vi "GUI Main Window.vi"() -> ()   [LabVIEW 2011]
doc: "Fast Orbit Feedback (FOFB) graphical user interface."
uses:
  Types Definitions/Type Configuration Loop Mode.ctl
  <vilib>/Platform/TimedLoop/XDataNode/timing_clust.ctl
  <vilib>/Platform/TimedLoop/XDataNode/nitl_modes.ctl
  <vilib>/Platform/TimedLoop/XDataNode/wakeup.ctl
  Types Definitions/Type Diagnostics Sample.ctl
  Types Definitions/Type Diagnostics Data.ctl
  Types Definitions/Type CPU Loads Array.ctl
  Types Definitions/Type CPU Loads.ctl
  Types Definitions/Type Monitoring Sample.ctl
  Types Definitions/Type FOFB Parameters.ctl
  Types Definitions/Type Network Configuration.ctl
  Types Definitions/Type FA Configuration.ctl
  Types Definitions/Type Response Matrix Measurement Configuration.ctl
  Types Definitions/Type Correction Algorithm Configuration.ctl
  Types Definitions/Type Acquisition Network Configuration.ctl
  Types Definitions/Type Actuation Network Configuration.ctl
  Types Definitions/Type BPM or PS Selector.ctl
  <vilib>/Analysis/5stat.llb/RMS (DBL).vi
  GUI Monitoring Graph Selection Window.vi
  <vilib>/Platform/TimedLoop/XDataNode/XDataNode.xnode
  <vilib>/Platform/TimedLoop/XDataNode/XDNodeRunTimeDep.lvlib
  File VIs.lvlib
  Type Definitions.lvlib
  Third Party/bean/bean.lvlib
  User Interface Window VIs.lvlib
  User Interface VIs.lvlib
  XML VIs.lvlib
  Filter VIs.lvlib
  <vilib>/Analysis/NI_AALPro.lvlib
panel:
  out "error out":errorcluster
  out "Connected":bool
  in  "Open Computer Performance":bool
  in  "Open BPM RMS/Min/Max Monitoring Graph":bool
  out "Orbit Path":path caption="Endereço da Órbita de Referência"
  in  "Open Configuration GUI":bool
  in  "Max Scale Y":dbl=1.0 min=0.001 max=20.0 format="%6.3g"
  in  "Max Scale X":dbl=1.0 min=0.001 max=20.0 format="%6.3g"
  in  "Auto-Scale":bool
  in  "Open BPM-PS Monitoring Graph":bool
  out "Reference Orbit":dbl[](array[numeric])
  in  "Orbit Source":enum32{"Zero", "From File", "Current Orbit"}(radio)
  out "Current Orbit":dbl[](array[numeric])
  out "Operation Mode (Controller to GUI)":T1(ring) caption="Modo de Operação"
  in  "Send Orbit":bool
  out "Min Y @":string="AMP05A" caption="@"
  out "MaxY @":string="AMP05A" caption="@"
  out "RMS Y":dbl=-1.1111 caption="RMS =" format="%#.4g"
  out "Min Y":dbl=-1.2564 caption="Min =" format="%#.4g"
  out "Max. Y":dbl=1.1111 caption="Max =" format="%#.4g"
  out "Min X @":string="AMP01A" caption="@"
  out "Max X @":string="AMP01A" caption="@"
  out "RMS X":dbl=21.1111 caption="RMS =" format="%#.4g"
  out "Min X":dbl=1.1111 caption="Min =" format="%#.4g"
  out "Max. X":dbl=1.1111 caption="Max =" format="%#.4g"
  out "Horizontal":cluster{i32, dbl}[](graph)
  out "Vertical":cluster{i32, dbl}[](graph)
  in  "Save Orbit":bool
  # "Órbita de Referência Local"
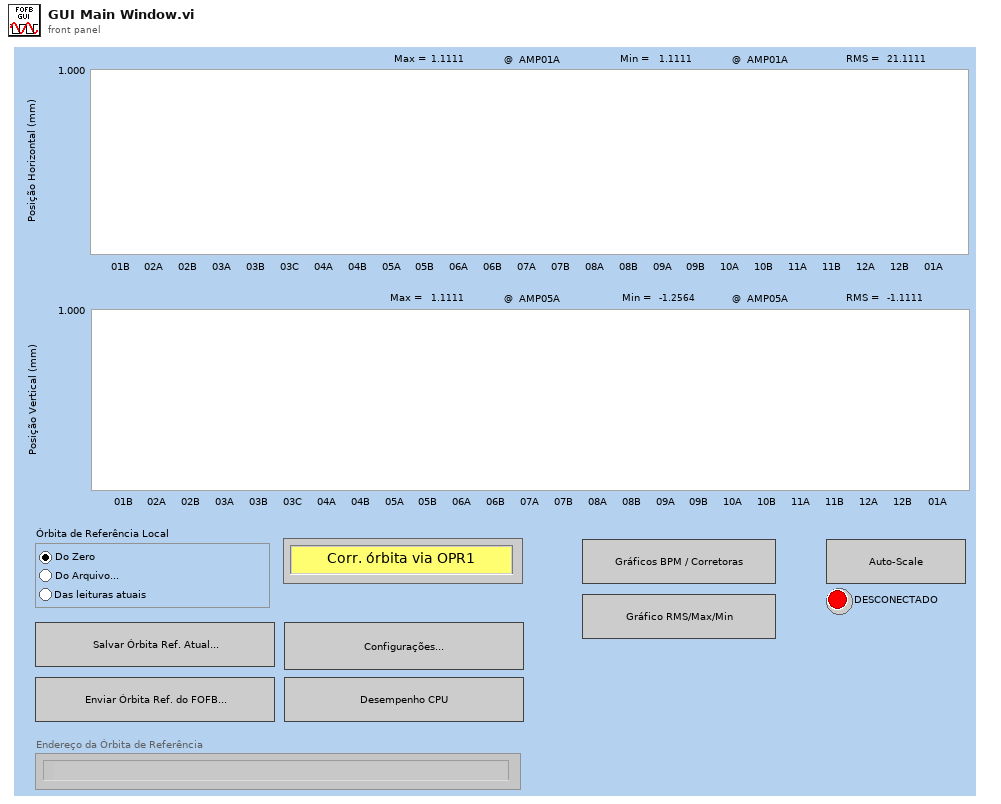
[diagram p1: front panel]
types:
  T1 = enum16{"Corr. órbita via OPR1", "Corr. órbita via FOFB", "Medida de Matriz Resposta"}
  T2 = enum8{"Enabled", "Disabled", "Disabled and Grayed Out"}
  T3 = typedef "Type Definitions.lvlib/Type Configuration Loop Mode.ctl" = enum8{"Operation Mode", "Request FOFB Parameters", "Send New FOFB Parameters", "Send Reference Orbit", "Request Response Matrix List Folder"}
  T4 = typedef "XDNodeRunTimeDep.lvlib/timing_clust.ctl" = cluster{"Expected End [f-1]":u64, "Actual End [f-1]":u64, "Finished Late? [f-1]":bool, "Expected End [i-1]":u64, "Actual End [i-1]":u64, "Finished Late? [i-1]":bool, "Expected Start [i]":u64, "Actual Start [i]":u64, "Expected Start [f]":u64, "Actual Start [f]":u64, "Source Name":string, "Structure Name":string, "Period":i64, "Deadline":i64, "Offset":i64, "Start":i64, "Priority":i32, "Timeout":i32, "Mode":T5, "Wakeup Reason":T6, "Error":errorcluster, "Source Type":string, "Secondary Source Type":string, "Global End Time":u64, "Global Start Time":u64, "Frame Duration":u64, "Iteration Duration":u64, "Assigned CPU":i32, "I/O Scan Engine Mode":u32}
  T5 = typedef "XDNodeRunTimeDep.lvlib/nitl_modes.ctl" = enum32{"No Change", "Process missed periods, maintain original phase", "Discard missed periods, maintain original phase", "Process missed periods, ignore original phase", "Discard missed periods, ignore original phase"}
  T6 = typedef "XDNodeRunTimeDep.lvlib/wakeup.ctl" = enum32{"Normal", "Aborted", "Asynchronous wakeup", "Timing source error", "Timed loop error", "Timeout"}
  T7 = enum32{"Invalid", "Standard", "Closed", "Hidden", "Minimized", "Maximized"}
  T8 = typedef "Type Definitions.lvlib/Type BPM or PS Selector.ctl" = cluster{"Name":string, "Active":bool}
  T9 = typedef "Type Definitions.lvlib/Type Diagnostics Sample.ctl" = cluster{"Timestamp":timestamp, "Diagnostics Data":T10}
  T10 = typedef "Type Definitions.lvlib/Type Diagnostics Data.ctl" = cluster{"Time-Critical Loop Missed Iterations":u32, "Time-Critical Loop Execution Time (usec)":u32, "FA Buffer Usage":u32, "Available Memory (bytes)":u32, "CPU Loads Array":T11}
  T11 = typedef "Type Definitions.lvlib/Type CPU Loads Array.ctl" = T12[]
  T12 = typedef "Type Definitions.lvlib/Type CPU Loads.ctl" = cluster{"Total (%)":dbl, "Time Critical (%)":dbl, "Timed Structures (%)":dbl, "High (%)":dbl, "Above Normal (%)":dbl, "Normal (%)":dbl, "Background (%)":dbl, "Idle (%)":dbl, "ISR (%)":dbl}
  T13 = enum16{"open", "open or create", "create or replace", "create", "open (read-only)"}
  T14 = typedef "Type Definitions.lvlib/Type FOFB GUI.ctl" = cluster{"Response Matrix List Folder Notifier":refnum<notifier>, "Send Reference Orbit Notifier":refnum<notifier>, "FOFB Parameters Notifier":refnum<notifier>, "Configuration Loop Mode Notifier":refnum<notifier>, "Stop VIs Notifier":refnum<notifier>, "GUI Configuration Notifier":refnum<notifier>, "Monitoring Data Notifier":refnum<queue>, "Performance Monitoring Data Notifier":refnum<queue>, "BPM / PS Monitoring Data Notifiers":refnum<queue>[], "Load Orbit Notifier":refnum<notifier>, "RMS Monitoring Data Queue":refnum<queue>, "GUI-Controller Connected Queue":refnum<queue>}
  T15 = typedef "Type Definitions.lvlib/Type FOFB Parameters.ctl" = cluster{"Network":T16, "Fast Acquisition":T17, "Response Matrix Measurement":T18, "Correction Algorithm":T19, "Acquisition Network":T20, "Actuation Network":T21}
  T16 = typedef "Type Definitions.lvlib/Type Network Configuration.ctl" = cluster{"FOFB Controller IP":string, "LNLS Control Network IP":string, "LNLS Control Network Power Supplies TCP Port":u16, "LNLS Control Network FOFB Configuration TCP Port":u16, "Data Server TCP Port":u16, "Monitoring Data TCP Port":u16, "Configuration GUI TCP Port":u16, "TCP Listening Timeout":i32}
  T17 = typedef "Type Definitions.lvlib/Type FA Configuration.ctl" = cluster{"Acquisition Period":u32, "Data Buffer Size":u32, "Monitoring Period":u32}
  T18 = typedef "Type Definitions.lvlib/Type Response Matrix Measurement Configuration.ctl" = cluster{"Step Amplitude":dbl, "Time Between Steps":u32, "Step Duration":u32, "Number of Averages":u32}
  T19 = typedef "Type Definitions.lvlib/Type Correction Algorithm Configuration.ctl" = cluster{"Correction Period":u32, "Reference Orbit Path":path, "Response Matrix Path":path, "Correction Matrix Path":path, "Horizontal Correction Factor":dbl, "Vertical Correction Factor":dbl, "Beam Current FOFB Threshold":dbl, "Decouple H-V":bool, "Use Additional BPM LPF":bool, "BPM LPF Cutoff":dbl}
  T20 = typedef "Type Definitions.lvlib/Type Acquisition Network Configuration.ctl" = cluster{"Chassis Name":string, "Variables":cluster{"Variable Name":string, "Matrix Order":u32, "Location":dbl, "Plane":enum8{"H", "V"}, "On Correction":bool}[]}[]
  T21 = typedef "Type Definitions.lvlib/Type Actuation Network Configuration.ctl" = cluster{"Chassis Name":string, "Variables":cluster{"Variable Name":string, "Matrix Order":u32, "RMM Step Factor":dbl, "Plane":enum8{"H", "V"}, "On Correction":bool, "Kc":dbl, "Ti":dbl, "Td":dbl}[]}[]
  T22 = typedef "Type Definitions.lvlib/Type Monitoring Sample.ctl" = cluster{"Timestamp":timestamp, "Sample":dbl[]}
  T23 = typedef "Type Definitions.lvlib/Type Monitoring Data.ctl" = cluster{"Timestamp":timestamp, "BPM Readings":dbl[], "PS Readings":dbl[], "PS FOFB Setpoints":dbl[], "PS Status per Rack":u8[], "PS ON-OFF per Rack":u8[], "Operation Mode":enum16{"Idle Mode", "Error Mode", "Manual Mode", "FOFB Mode", "RMM Mode"}, "Diagnostics Data":T10, "Controller Status Table":i32[]}
  T24 = enum16{"Idle Mode", "Error Mode", "Manual Mode", "FOFB Mode", "RMM Mode"}
  T25 = typedef "LVDateTimeRec.ctl" = cluster{"fractional second":dbl, "second":i32, "minute":i32, "hour":i32, "day of month":i32, "month":i32, "year":i32, "day of week":i32, "day of year":i32, "DST":i32}
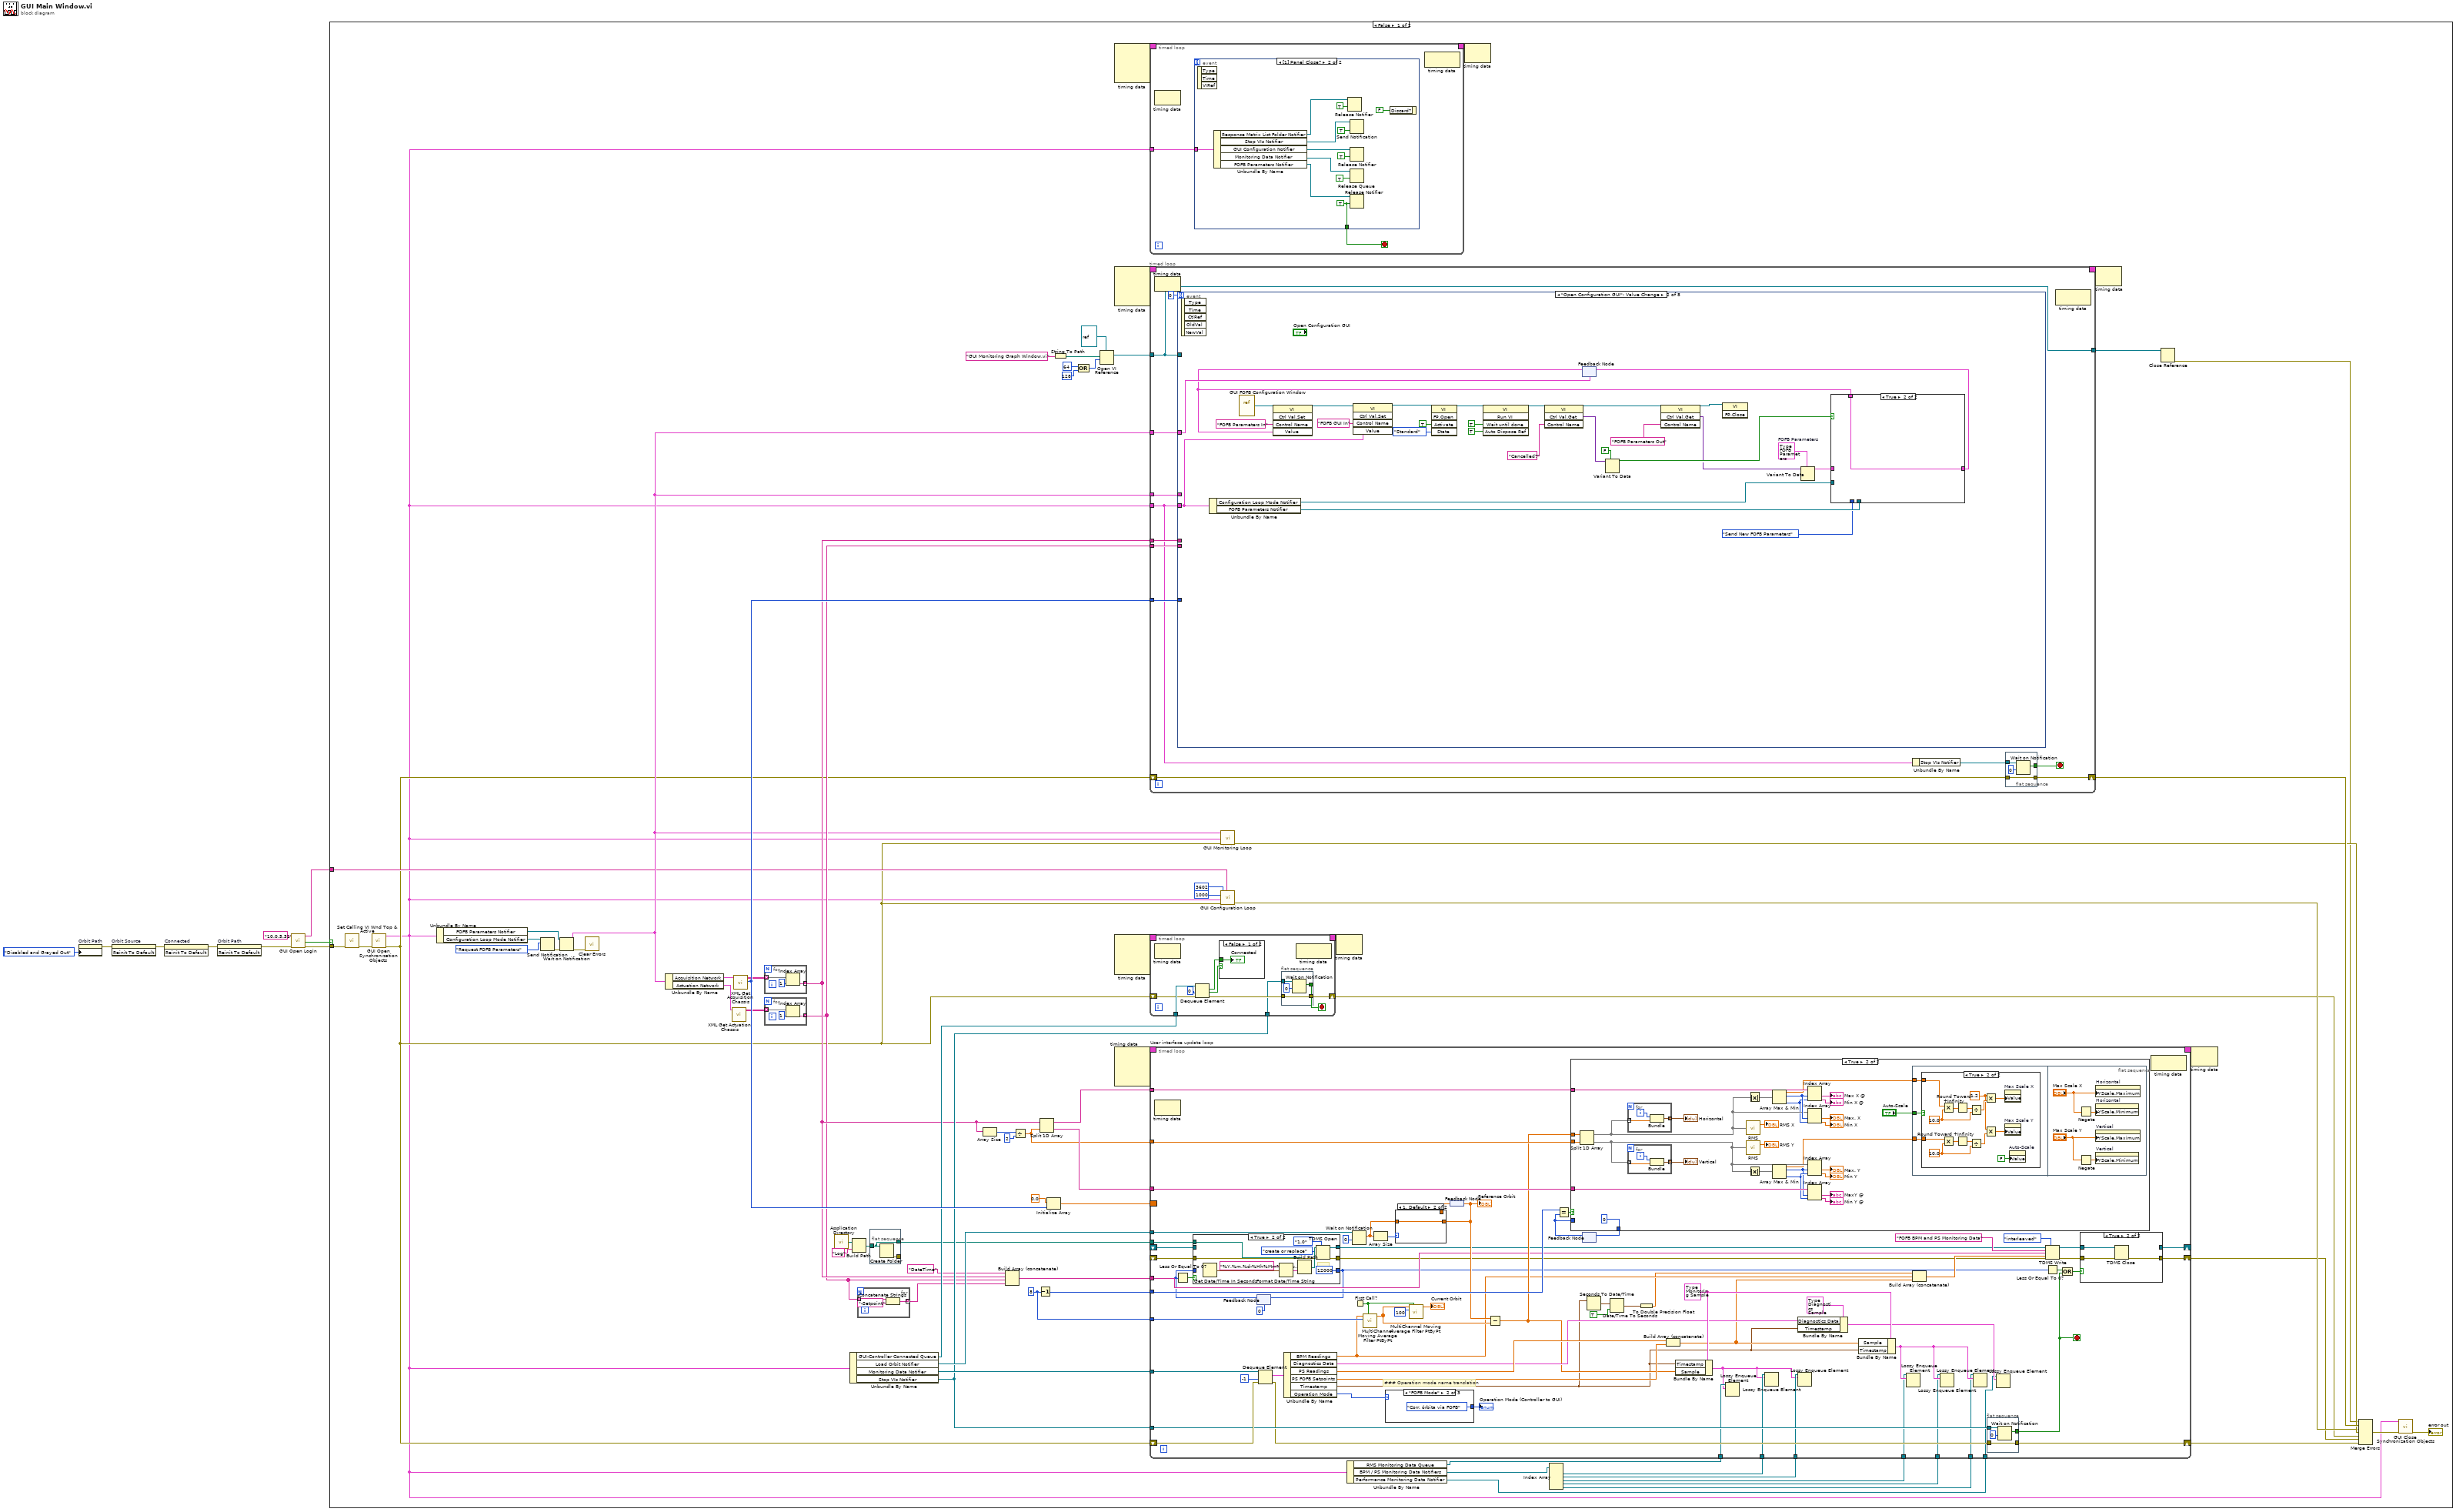
[diagram p0: block diagram]
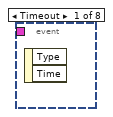
[diagram p3: hidden frame]
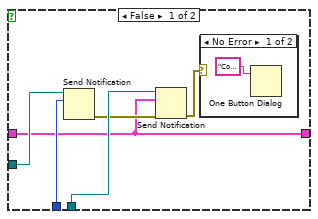
[diagram p4: hidden frame]
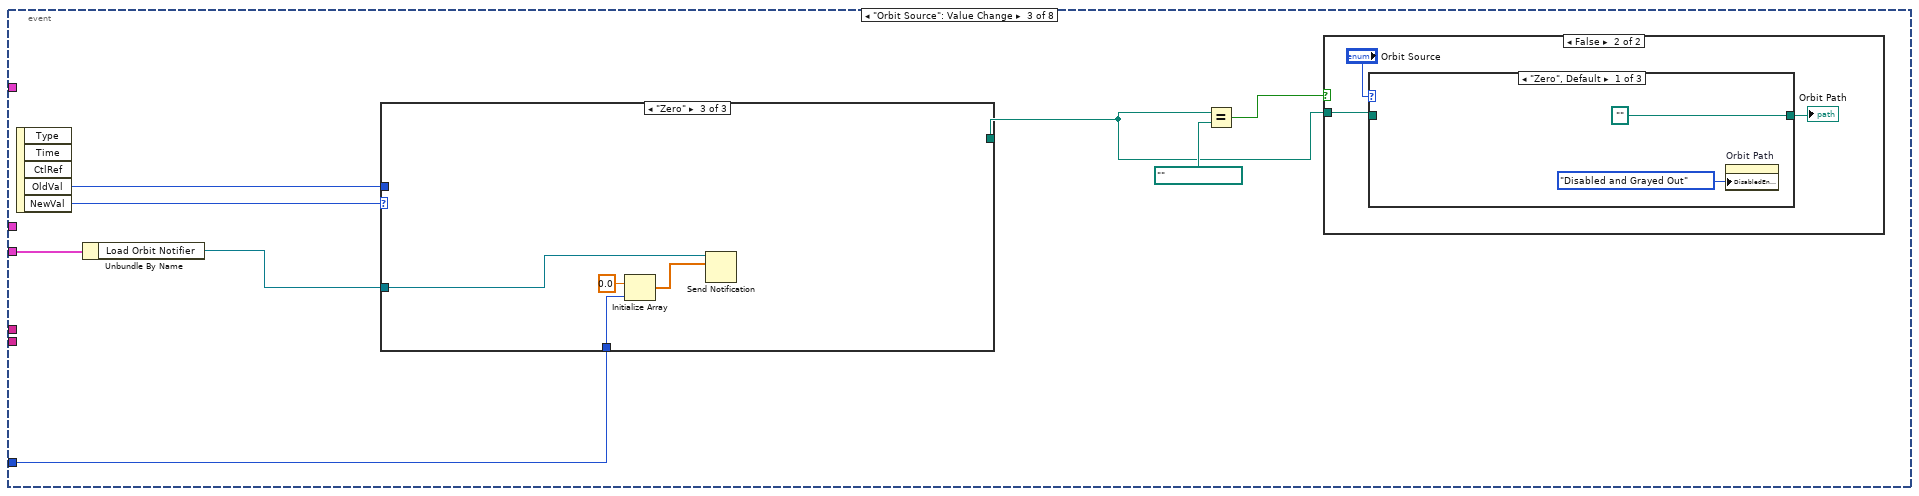
[diagram p6: hidden frame]
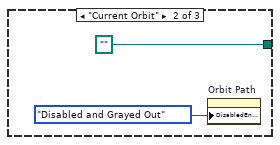
[diagram p8: hidden frame]
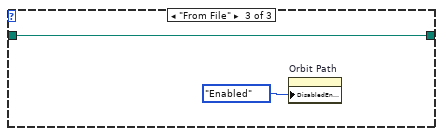
[diagram p9: hidden frame]
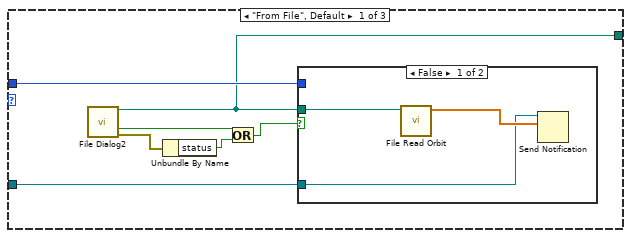
[diagram p10: hidden frame]
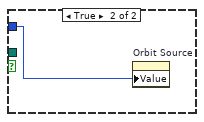
[diagram p11: hidden frame]
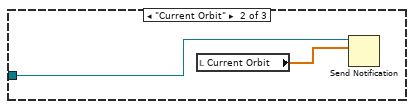
[diagram p12: hidden frame]
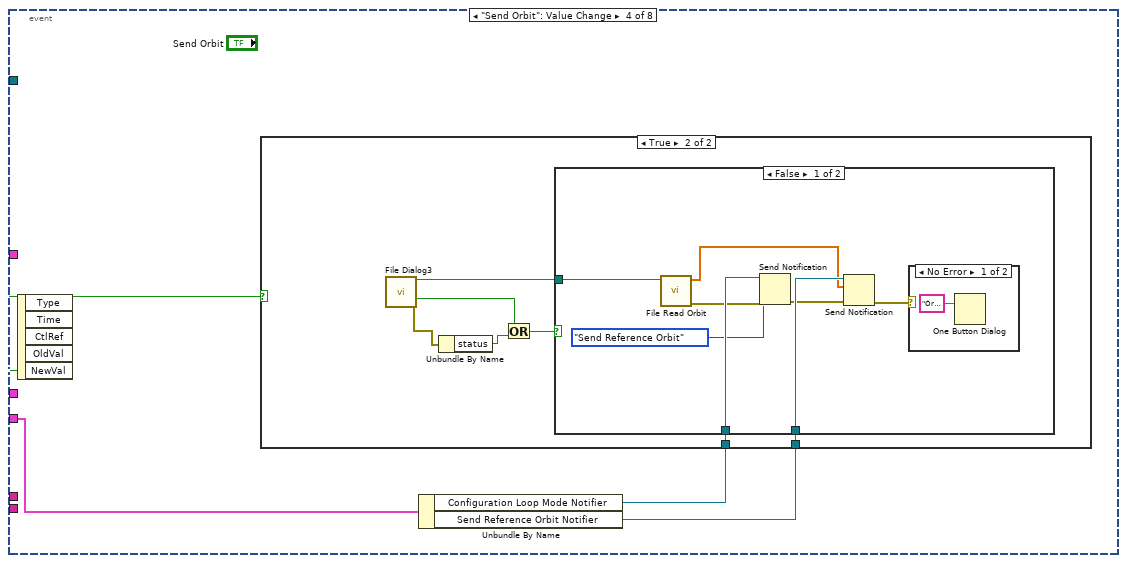
[diagram p13: hidden frame]
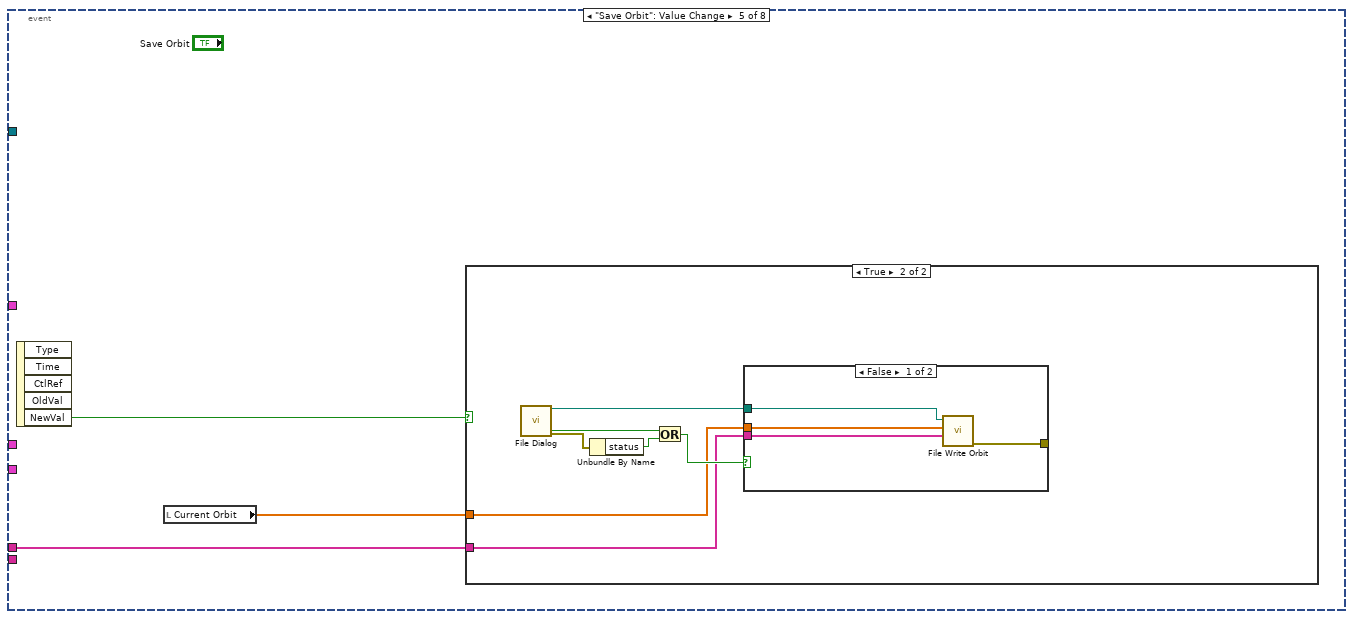
[diagram p17: hidden frame]
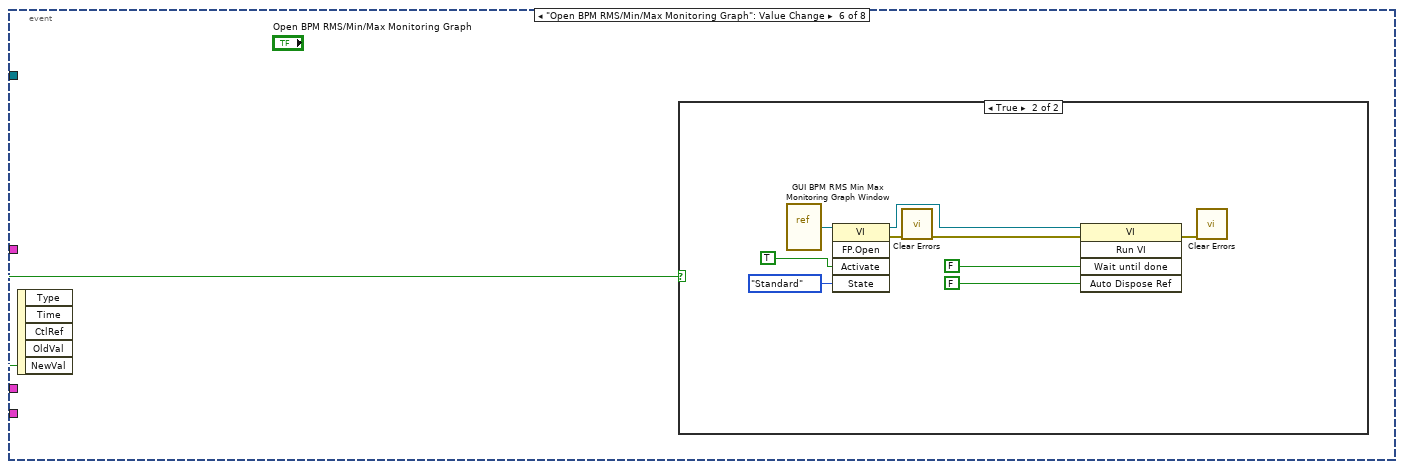
[diagram p20: hidden frame]
diagram:
  (unwired) T2."Disabled and Grayed Out" ("Disabled")
  n1 = property on="Orbit Path" class="Path"("DisabledEnum"=T2."Disabled and Grayed Out" ("Disabled")) -> (error out=w8:errorcluster)  [unwired: 2 in, 1 out]
  n2 = invoke on="Orbit Source" class="RadioBtnsControl (strict)" method="Reinit To Default"(error in=w8) -> (error out=w7:errorcluster)  [unwired: 2 in, 2 out]
  n3 = invoke on="Connected" class="Bool (strict)" method="Reinit To Default"(error in=w7) -> (error out=w6:errorcluster)  [unwired: 2 in, 2 out]
  n4 = invoke on="Orbit Path" class="Path" method="Reinit To Default"(error in=w6) -> (error out=w5:errorcluster)  [unwired: 2 in, 2 out]
  n5 = call "GUI Open Login.vi"("error in (no error)"=w5, "Controller IP Address in"="10.0.5.31" ("FOFB-Controller IP Address in")) -> ("error out"=w2:errorcluster, "Cancelled?"=w1:bool, "Controller IP Address out"=w3:string)  [unwired: 6 in, 1 out]
  n6 = case shown="False" w1 {
    tunnel: w2 -> [w13 _]
    tunnel: w3 -> [w14 _]
    frame False {
      w63 = u32 8 ("Number of Averages")
      n7 = call "Set Calling VI Wnd Top & Active.vi"("Error In"=w13) -> ("Error Out"=w11:errorcluster)  [unwired: 10 in]
      n8 = call "GUI Open Synchronization Objects.vi"("error in (no error)"=w11) -> ("error out"=w12:errorcluster, "FOFB GUI"=w10:T14)  [unwired: 9 in]
      n9 = Unbundle By Name(w10) -> ("FOFB Parameters Notifier"=w20:refnum<notifier>, "Configuration Loop Mode Notifier"=w21:refnum<notifier>)
      n10 = Send Notification(notification=Type_Configuration_Loop_Mode."Request FOFB Parameters", notifier=w21) -> (error out=w24:errorcluster)  [unwired: 1 in, 1 out]
      n11 = Wait on Notification(notifier=w20, error in (no error)=w24) -> (notification=w15:T15, error out=w18:errorcluster)  [unwired: 2 in, 2 out]
      n12 = call <vilib>:"Clear Errors.vi"("error in (no error)"=w18) -> ()  [unwired: 6 in, 1 out]
      n13 = Unbundle By Name(w15) -> ("Acquisition Network"=w73:T20, "Actuation Network"=w72:T21)
      n14 = call "XML Get Actuation Chassis.vi"("Actuation Network"=w72) -> ("Actuation Variable Names"=w70:string[][])  [unwired: 3 in, 7 out]
      n15 = call "XML Get Acquisition Chassis.vi"("Acquisition Network"=w73) -> ("Number of BPM Readings"=w74:i32, "Acquisition Variable Names"=w71:string[][])  [unwired: 4 in, 5 out]
      n16 = for {
        tunnel: w71 -> [w528] mode=indexing
        tunnel: [w527] -> w34 mode=indexing
        n17 = Index Array(array=w528, index=1) -> (element=w527:string)
      }
      n18 = for {
        tunnel: w70 -> [w525] mode=indexing
        tunnel: [w524] -> w32 mode=indexing
        n19 = Index Array(array=w525, index=1) -> (element=w524:string)
      }
      n20 = call <vilib>:"Application Directory.vi"() -> ("Application Directory"=w28:path)
      n21 = Unbundle By Name(w10) -> ("GUI-Controller Connected Queue"=w52:refnum<queue>, "Load Orbit Notifier"=w57:refnum<notifier>, "Monitoring Data Notifier"=w58:refnum<queue>, "Stop VIs Notifier"=w51:refnum<notifier>)
      n22 = Build Path(base path=w28, name or relative path="Log") -> (appended path=w26:path)
      n23 = for {
        tunnel: w32 -> [w87] mode=indexing
        tunnel: [w86] -> w31 mode=indexing
        n24 = Concatenate Strings(w87, "-Setpoint" ("string")) -> (w86:string)
      }
      n25 = flat-sequence {
        tunnel: w26 -> [w84]
        tunnel: [w84] -> w25
        tunnel: [w83] -> _
        frame #0 {
          n26 = Create Folder(path (use dialog)=w84) -> (error out=w83:errorcluster)  [unwired: 2 in, 2 out]
        }
      }
      n27 = Array Size(array=w34) -> (size(s)=w65:i32)
      n28 = Build Array (concatenate)("DateTime" ("name or relative path"), w34, w32, w31) -> (w33:string[])
      n29 = Divide(x=w65, y=2) -> (x/y=w48:dbl)
      n30 = Decrement(x=w63) -> (x-1=w62:u32)
      n31 = Split 1D Array(array=w34, index=w48) -> (first subarray=w50:string[], second subarray=w49:string[])
      n32 = Initialize Array(0.0 ("element"), w74) -> (w60:dbl[])
      n33 = String To Path(string="GUI Monitoring Graph Window.vi") -> (path=w36:path)
      n34 = Compound Arithmetic op=OR(64 ("options"), 128 ("options")) -> (w40:i32)
      n35 = Open VI Reference(type specifier VI Refnum (for type only)=refnum<vi> refnum, vi path=w36, options=w40) -> (vi reference=w59:refnum<vi>)  [unwired: 3 in, 1 out]
      n36 = node-c288() -> (w82:T4)  [unwired: 4 in]
      n37 = node-c288() -> (w78:T4)  [unwired: 4 in]
      n38 = node-c288() -> (w76:T4)  [unwired: 4 in]
      n39 = node-c288() -> (w80:T4)  [unwired: 4 in]
      n40 = timed-loop {
        timing: w82 -> [_]
        timing-out: [_] -> w81
        tunnel: w10 -> [w531]
        stop <- w530 stop-if-true
        n41 = node-c288() -> ()  [unwired: 1 in, 1 out]
        n42 = event shown="[1] Panel Close?" {
          selector: _ -> [_ _]
          dyn-events: _ -> [_ _]
          timeout: _ -> [_ _]
          tunnel: w531 -> [_ w535]
          tunnel: [_ w536] -> w530
          event Timeout {
            n43 = event-data() -> ()  [unwired: 1 in, 2 out]
          }
          event Panel Close? {
            w536 = TRUE ("force destroy? (F)")
            n44 = event-data() -> ()  [unwired: 1 in, 3 out]
            n45 = Unbundle By Name(w535) -> ("Response Matrix List Folder Notifier"=w533:refnum<notifier>, "Stop VIs Notifier"=w540:refnum<notifier>, "GUI Configuration Notifier"=w542:refnum<notifier>, "Monitoring Data Notifier"=w537:refnum<queue>, "FOFB Parameters Notifier"=w543:refnum<notifier>)
            n46 = Release Notifier(notifier=w533, force destroy? (F)=TRUE) -> ()  [unwired: 1 in, 3 out]
            n47 = Send Notification(notification=TRUE, notifier=w540) -> ()  [unwired: 1 in, 2 out]
            n48 = Release Notifier(notifier=w542, force destroy? (F)=TRUE) -> ()  [unwired: 1 in, 3 out]
            n49 = Release Queue(queue=w537, force destroy? (F)=TRUE) -> ()  [unwired: 1 in, 3 out]
            n50 = Release Notifier(notifier=w543, force destroy? (F)=w536) -> ()  [unwired: 1 in, 3 out]
            n51 = event-data("Discard?"=FALSE) -> ()  [unwired: 1 in, 1 out]
          }
        }
        n52 = node-c288() -> ()  [unwired: 1 in, 1 out]
      }
      n53 = timed-loop {
        tunnel: w34 -> [w117]
        tunnel: w74 -> [w116]
        tunnel: w32 -> [w115]
        timing: w78 -> [_]
        timing-out: [_] -> w77
        tunnel: w59 -> [w114]
        tunnel: [w114] -> w55
        shift-right: [w111] -> w69
        shift-left: w12 -> [w112]
        tunnel: w10 -> [w109]
        tunnel: w15 -> [w113]
        tunnel: w15 -> [w106]
        stop <- w110 stop-if-true
        n54 = node-c288() -> ()  [unwired: 1 in, 1 out]
        n55 = event shown="[1] \"Open Configuration GUI\": Value Change" {
          selector: _ -> [_ _ _ _ _ _ _ _]
          dyn-events: _ -> [_ _ _ _ _ _ _ _]
          timeout: 0 -> [_ _ _ _ _ _ _ _]
          tunnel: w117 -> [_ _ _ _ w215 _ w240 _]
          tunnel: w116 -> [_ _ w165 _ _ _ _ _]
          tunnel: w115 -> [_ _ _ _ _ _ w242 _]
          tunnel: w114 -> [_ _ _ _ _ _ w241 _]
          tunnel: w109 -> [_ w127 w160 w196 _ _ _ _]
          tunnel: w113 -> [_ _ _ _ _ _ _ _]
          tunnel: w106 -> [_ w125 _ _ _ _ _ _]
          event Timeout {
            n56 = event-data() -> ()  [unwired: 1 in, 2 out]
          }
          event "Open Configuration GUI": Value Change {
            w135 = T15 {"Network"={"FOFB Controller IP"="", "LNLS Control Network IP"="", "LNLS Control Network Power Supplies TCP Port"=0, "LNLS Control Network FOFB Configuration TCP Port"=0, "Data Server TCP Port"=0, "Monitoring Data TCP Port"=0, "Configuration GUI TCP Port"=0, "TCP Listening Timeout"=0}, "Fast Acquisition"={"Acquisition Period"=0, "Data Buffer Size"=0, "Monitoring Period"=0}, "Response Matrix Measurement"={"Step Amplitude"=0.0, "Time Between Steps"=0, "Step Duration"=0, "Number of Averages"=0}, "Correction Algorithm"={"Correction Period"=0, "Reference Orbit Path"=path "", "Response Matrix Path"=path "", "Correction Matrix Path"=path "", "Horizontal Correction Factor"=0.0, "Vertical Correction Factor"=0.0, "Beam Current FOFB Threshold"=0.0, "Decouple H-V"=FALSE, "Use Additional BPM LPF"=FALSE, "BPM LPF Cutoff"=0.0}, "Acquisition Network"=[], "Actuation Network"=[]}  # FOFB Parameters
            n57 = event-data() -> ()  [unwired: 1 in, 5 out]
            n58 = Unbundle By Name(w127) -> ("Configuration Loop Mode Notifier"=w128:refnum<notifier>, "FOFB Parameters Notifier"=w134:refnum<notifier>)
            n59 = vi-ref "GUI FOFB Configuration Window.vi"() -> (w140:refnum<vi>)
            n60 = feedback #1(w125) -> (w124:T15)
            n61 = invoke class="VI" method="Ctrl Val.Set"(reference=w140, "Control Name"="FOFB Parameters In", "Value"=w124) -> (reference out=w131:refnum<vi>)  [unwired: 2 in, 4 out]
            n62 = invoke class="VI" method="Ctrl Val.Set"(reference=w131, "Control Name"="FOFB GUI In", "Value"=w127) -> (reference out=w130:refnum<vi>)  [unwired: 2 in, 4 out]
            n63 = invoke class="VI" method="FP.Open"(reference=w130, "Activate"=TRUE ("Activate?"), "State"=T7."Standard") -> (reference out=w147:refnum<vi>)  [unwired: 2 in, 4 out]
            n64 = invoke class="VI" method="Run VI"(reference=w147, "Wait until done"=TRUE ("Wait Until Done"), "Auto Dispose Ref"=TRUE ("Auto Dispose Reference")) -> (reference out=w148:refnum<vi>)  [unwired: 2 in, 4 out]
            n65 = invoke class="VI" method="Ctrl Val.Get"(reference=w148, "Control Name"="Cancelled?") -> (reference out=w139:refnum<vi>, "Get Control Value Variant"=w142:variant)  [unwired: 2 in, 2 out]
            n66 = Variant To Data(type=FALSE ("Stop?"), Variant=w142) -> (data=w141:bool)  [unwired: 1 in, 1 out]
            n67 = invoke class="VI" method="Ctrl Val.Get"(reference=w139, "Control Name"="FOFB Parameters Out") -> (reference out=w138:refnum<vi>, "Get Control Value Variant"=w136:variant)  [unwired: 2 in, 2 out]
            n68 = invoke class="VI" method="FP.Close"(reference=w138) -> ()  [unwired: 2 in, 3 out]
            n69 = Variant To Data(type=w135, Variant=w136) -> (data=w133:T15)  [unwired: 1 in, 1 out]
            n70 = case shown="True" w141 {
              tunnel: w128 -> [w157 _]
              tunnel: w134 -> [w156 _]
              tunnel: w133 -> [w153 _]
              tunnel: [w153 w159] -> w126
              tunnel: Type_Configuration_Loop_Mode."Send New FOFB Parameters" ("notification") -> [w154 _]
              tunnel: w124 -> [_ w159]
              frame False {
                n71 = Send Notification(notification=w154, notifier=w157) -> (error out=w155:errorcluster)  [unwired: 1 in, 1 out]
                n72 = Send Notification(notification=w153, notifier=w156, error in (no error)=w155) -> (error out=w152:errorcluster)  [unwired: 1 out]
                n73 = case shown="No Error" w152 {
                  frame No Error {
                    n74 = One Button Dialog(message="Configurações alteradas com sucesso") -> ()  [unwired: 1 in, 1 out]
                  }
                  frame Error {
                  }
                }
              }
              frame True {
              }
            }
            n75 = feedback-in #1(w126) -> ()
          }
          event "Orbit Source": Value Change {
            n76 = event-data() -> ("OldVal"=w166:enum32{"Zero", "From File", "Current Orbit"}, "NewVal"=w167:enum32{"Zero", "From File", "Current Orbit"})  [unwired: 1 in, 3 out]
            n77 = Unbundle By Name(w160) -> ("Load Orbit Notifier"=w161:refnum<notifier>)
            n78 = case shown="\"Zero\"" w167 {
              tunnel: w161 -> [w180 w189 w193]
              tunnel: w166 -> [w179 _ _]
              tunnel: w165 -> [_ _ w192]
              tunnel: [w178 _ _] -> w163
              frame "From File", Default {
                n79 = call "File Dialog2"() -> ("selected path"=w178:path, "cancelled"=w177:bool, "error out"=w181:errorcluster)  [unwired: 12 in, 1 out]
                n80 = Unbundle By Name(w181) -> ("status"=w182:bool)
                n81 = Or(x=w177, y=w182) -> (x .or. y?=w183:bool)
                n82 = case shown="False" w183 {
                  tunnel: w178 -> [w186 _]
                  tunnel: w180 -> [w184 _]
                  tunnel: w179 -> [_ w187]
                  frame False {
                    n83 = call "File Read Orbit.vi"("file path (dialog if empty)"=w186) -> ("Orbit"=w185:dbl[])  [unwired: 8 in, 2 out]
                    n84 = Send Notification(notification=w185, notifier=w184) -> ()  [unwired: 1 in, 2 out]
                  }
                  frame True {
                    n85 = property on="Orbit Source" class="RadioBtnsControl (strict)"("Value"=w187) -> ()  [unwired: 2 in, 2 out]
                  }
                }
              }
              frame "Current Orbit" {
                n86 = local read "Current Orbit"() -> (w188:dbl[])
                n87 = Send Notification(notification=w188, notifier=w189) -> ()  [unwired: 1 in, 2 out]
              }
              frame "Zero" {
                n88 = Initialize Array(0.0 ("element"), w192) -> (w191:dbl[])
                n89 = Send Notification(notification=w191, notifier=w193) -> ()  [unwired: 1 in, 2 out]
              }
            }
            n90 = Equal?(x=w163, y=path "" ("Orbit Path")) -> (x = y?=w162:bool)
            n91 = case shown="False" w162 {
              tunnel: w163 -> [_ w168]
              frame True {
              }
              frame False {
                n92 = case shown="\"Zero\", Default" "Orbit Source" {
                  tunnel: w168 -> [_ _ w176]
                  tunnel: [path "" ("selected path") path "" ("selected path") w176] -> w170
                  frame "Zero", Default {
                    n93 = property on="Orbit Path" class="Path"("DisabledEnum"=T2."Disabled and Grayed Out" ("Disabled")) -> ()  [unwired: 2 in, 2 out]
                  }
                  frame "Current Orbit" {
                    n94 = property on="Orbit Path" class="Path"("DisabledEnum"=T2."Disabled and Grayed Out" ("Disabled")) -> ()  [unwired: 2 in, 2 out]
                  }
                  frame "From File" {
                    n95 = property on="Orbit Path" class="Path"("DisabledEnum"=T2."Enabled" ("Disabled")) -> ()  [unwired: 2 in, 2 out]
                  }
                }
                "Orbit Path" <- w170
              }
            }
          }
          event "Send Orbit": Value Change {
            n96 = event-data() -> ("NewVal"=w197:bool)  [unwired: 1 in, 4 out]
            n97 = Unbundle By Name(w196) -> ("Configuration Loop Mode Notifier"=w195:refnum<notifier>, "Send Reference Orbit Notifier"=w194:refnum<notifier>)
            n98 = case shown="True" w197 {
              tunnel: w195 -> [_ w199]
              tunnel: w194 -> [_ w198]
              frame False {
              }
              frame True {
                n99 = call "File Dialog3"() -> ("selected path"=w200:path, "cancelled"=w204:bool, "error out"=w202:errorcluster)  [unwired: 12 in, 1 out]
                n100 = Unbundle By Name(w202) -> ("status"=w203:bool)
                n101 = Or(x=w204, y=w203) -> (x .or. y?=w201:bool)
                n102 = case shown="False" w201 {
                  tunnel: w200 -> [w212 _]
                  tunnel: w199 -> [w211 _]
                  tunnel: w198 -> [w210 _]
                  frame False {
                    n103 = call "File Read Orbit.vi"("file path (dialog if empty)"=w212) -> ("error out"=w209:errorcluster, "Orbit"=w206:dbl[])  [unwired: 8 in, 1 out]
                    n104 = Send Notification(notification=Type_Configuration_Loop_Mode."Send Reference Orbit", notifier=w211, error in (no error)=w209) -> (error out=w208:errorcluster)  [unwired: 1 out]
                    n105 = Send Notification(notification=w206, notifier=w210, error in (no error)=w208) -> (error out=w205:errorcluster)  [unwired: 1 out]
                    n106 = case shown="No Error" w205 {
                      frame No Error {
                        n107 = One Button Dialog(message="Órbita de referência alterada com sucesso") -> ()  [unwired: 1 in, 1 out]
                      }
                      frame Error {
                      }
                    }
                  }
                  frame True {
                  }
                }
              }
            }
          }
          event "Save Orbit": Value Change {
            n108 = event-data() -> ("NewVal"=w216:bool)  [unwired: 1 in, 4 out]
            n109 = local read "Current Orbit"() -> (w214:dbl[])
            n110 = case shown="True" w216 {
              tunnel: w215 -> [_ w218]
              tunnel: w214 -> [_ w217]
              frame False {
              }
              frame True {
                n111 = call "File Dialog"() -> ("selected path"=w219:path, "cancelled"=w221:bool, "error out"=w223:errorcluster)  [unwired: 12 in, 1 out]
                n112 = Unbundle By Name(w223) -> ("status"=w222:bool)
                n113 = Or(x=w221, y=w222) -> (x .or. y?=w220:bool)
                n114 = case shown="False" w220 {
                  tunnel: w219 -> [w227 _]
                  tunnel: w218 -> [w226 _]
                  tunnel: w217 -> [w225 _]
                  tunnel: [w224 _] -> _
                  frame False {
                    n115 = call "File Write Orbit.vi"("BPM Reading Names"=w226, "Orbit"=w225, "file path (dialog if empty)"=w227) -> ("error out"=w224:errorcluster)  [unwired: 7 in]
                  }
                  frame True {
                  }
                }
              }
            }
          }
          event "Open BPM RMS/Min/Max Monitoring Graph": Value Change {
            n116 = event-data() -> ("NewVal"=w228:bool)  [unwired: 1 in, 4 out]
            n117 = case shown="True" w228 {
              frame False {
              }
              frame True {
                n118 = vi-ref "GUI BPM RMS Min Max Monitoring Graph Window.vi"() -> (w233:refnum<vi>)
                n119 = invoke class="VI" method="FP.Open"(reference=w233, "Activate"=TRUE ("Activate?"), "State"=T7."Standard") -> (reference out=w232:refnum<vi>, error out=w230:errorcluster)  [unwired: 2 in, 3 out]
                n120 = call <vilib>:"Clear Errors.vi"("error in (no error)"=w230) -> ("error out"=w231:errorcluster)  [unwired: 6 in]
                n121 = invoke class="VI" method="Run VI"(reference=w232, error in=w231, "Wait until done"=FALSE ("Wait Until Done"), "Auto Dispose Ref"=FALSE ("Auto Dispose Reference")) -> (error out=w229:errorcluster)  [unwired: 1 in, 4 out]
                n122 = call <vilib>:"Clear Errors.vi"("error in (no error)"=w229) -> ()  [unwired: 6 in, 1 out]
              }
            }
          }
          event "Open BPM-PS Monitoring Graph": Value Change {
            n123 = event-data() -> ()  [unwired: 1 in, 5 out]
            n124 = vi-ref "User Interface Window VIs.lvlib:GUI Monitoring Graph Selection Window.vi"() -> (w239:refnum<vi>)
            n125 = invoke class="VI" method="FP.Open"(reference=w239, "Activate"=TRUE ("Activate?"), "State"=T7."Standard") -> (reference out=w238:refnum<vi>)  [unwired: 2 in, 4 out]
            n126 = invoke class="VI" method="Run VI"(reference=w238) -> (reference out=w248:refnum<vi>)  [unwired: 4 in, 4 out]
            n127 = invoke class="VI" method="Ctrl Val.Get"(reference=w248, "Control Name"="Graph Selector Out") -> (reference out=w243:refnum<vi>, "Get Control Value Variant"=w250:variant)  [unwired: 2 in, 2 out]
            n128 = Variant To Data(type=T8[] [{"Name"="", "Active"=FALSE}] ("BPM Graph Selector Horizontal"), Variant=w250) -> (data=w244:T8[])  [unwired: 1 in, 1 out]
            n129 = invoke class="VI" method="Ctrl Val.Get"(reference=w243, "Control Name"="Start plotting?") -> (reference out=w255:refnum<vi>, "Get Control Value Variant"=w246:variant)  [unwired: 2 in, 2 out]
            n130 = Variant To Data(type=TRUE, Variant=w246) -> (data=w245:bool)  [unwired: 1 in, 1 out]
            n131 = case shown="True" w245 {
              tunnel: w244 -> [_ w260]
              tunnel: w241 -> [_ w259]
              tunnel: w242 -> [_ w258]
              tunnel: w240 -> [_ w257]
              frame False {
              }
              frame True {
                n132 = for {
                  tunnel: w260 -> [w351] mode=indexing
                  tunnel: [w350] -> w256 mode=indexing
                  n133 = Unbundle By Name(w351) -> ("Active"=w350:bool)
                }
                n134 = for {
                  tunnel: w256 -> [w264] mode=indexing
                  tunnel: w259 -> [w265]
                  tunnel: w258 -> [w262]
                  tunnel: w257 -> [w261]
                  i -> [w263]
                  n135 = case shown="0, Default" w263 {
                    tunnel: w265 -> [w268 w284 w300 w317 w334]
                    tunnel: w264 -> [w267 w283 w299 w316 w333]
                    tunnel: w262 -> [w266 w282 w298 w315 w332]
                    tunnel: w261 -> [_ _ _ w314 w331]
                    frame 2 {
                      n136 = case shown="True" w267 {
                        tunnel: w268 -> [_ w278]
                        tunnel: w266 -> [_ w274]
                        frame False {
                        }
                        frame True {
                          n137 = call "GUI PS Group Indexes.vi"("PS Group"=enum16{"ACH", "ACV", "ALV"}."ACH") -> ("Indexes"=w270:i32[])  [unwired: 10 in]
                          n138 = call "GUI Build PS Vector.vi"("PS Indexes in"=w270) -> ("PS Indexes out"=w271:i32[])  [unwired: 10 in]
                          n139 = for {
                            tunnel: w274 -> [w279]
                            tunnel: w270 -> [w281] mode=indexing
                            tunnel: [w280] -> w273 mode=indexing
                            n140 = Index Array(array=w279, index=w281) -> (element=w280:string)
                          }
                          n141 = call-by-ref "Start Asynchronous Call"(reference=w278, "Graph Unit"="Corrente (A)", "Window Title"="FOFB - Gráfico Grupo ACH", "BPM?"=FALSE, "Monitoring Queue Name"="ACH Monitoring Data" ("Window Title"), "Selected Readings"=w271, "Variable Names"=w273) -> ()  [unwired: 7 in, 2 out]
                        }
                      }
                    }
                    frame 3 {
                      n142 = case shown="True" w283 {
                        tunnel: w284 -> [_ w294]
                        tunnel: w282 -> [_ w290]
                        frame False {
                        }
                        frame True {
                          n143 = call "GUI PS Group Indexes.vi"("PS Group"=enum16{"ACH", "ACV", "ALV"}."ACV") -> ("Indexes"=w285:i32[])  [unwired: 10 in]
                          n144 = call "GUI Build PS Vector.vi"("PS Indexes in"=w285) -> ("PS Indexes out"=w287:i32[])  [unwired: 10 in]
                          n145 = for {
                            tunnel: w290 -> [w295]
                            tunnel: w285 -> [w297] mode=indexing
                            tunnel: [w296] -> w289 mode=indexing
                            n146 = Index Array(array=w295, index=w297) -> (element=w296:string)
                          }
                          n147 = call-by-ref "Start Asynchronous Call"(reference=w294, "Graph Unit"="Corrente (A)", "Window Title"="FOFB - Gráfico Grupo ACV", "BPM?"=FALSE, "Monitoring Queue Name"="ACV Monitoring Data" ("Window Title"), "Selected Readings"=w287, "Variable Names"=w289) -> ()  [unwired: 7 in, 2 out]
                        }
                      }
                    }
                    frame 4 {
                      n148 = case shown="True" w299 {
                        tunnel: w300 -> [_ w310]
                        tunnel: w298 -> [_ w306]
                        frame False {
                        }
                        frame True {
                          n149 = call "GUI PS Group Indexes.vi"("PS Group"=enum16{"ACH", "ACV", "ALV"}."ALV") -> ("Indexes"=w302:i32[])  [unwired: 10 in]
                          n150 = call "GUI Build PS Vector.vi"("PS Indexes in"=w302) -> ("PS Indexes out"=w303:i32[])  [unwired: 10 in]
                          n151 = for {
                            tunnel: w306 -> [w311]
                            tunnel: w302 -> [w313] mode=indexing
                            tunnel: [w312] -> w305 mode=indexing
                            n152 = Index Array(array=w311, index=w313) -> (element=w312:string)
                          }
                          n153 = call-by-ref "Start Asynchronous Call"(reference=w310, "Graph Unit"="Corrente (A)", "Window Title"="FOFB - Gráfico Grupo ALV", "BPM?"=FALSE, "Monitoring Queue Name"="ALV Monitoring Data" ("Window Title"), "Selected Readings"=w303, "Variable Names"=w305) -> ()  [unwired: 7 in, 2 out]
                        }
                      }
                    }
                    frame 0, Default {
                      n154 = case shown="True" w316 {
                        tunnel: w317 -> [_ w326]
                        tunnel: w315 -> [_ _]
                        tunnel: w314 -> [_ w319]
                        frame False {
                        }
                        frame True {
                          n155 = for {
                            N: 25 -> [_]
                            tunnel: [w327] -> w320 mode=indexing
                            i -> [w327]
                          }
                          n156 = for {
                            tunnel: w319 -> [w328]
                            tunnel: w320 -> [w330] mode=indexing
                            tunnel: [w329] -> w322 mode=indexing
                            n157 = Index Array(array=w328, index=w330) -> (element=w329:string)
                          }
                          n158 = call-by-ref "Start Asynchronous Call"(reference=w326, "Graph Unit"="Amplitude (mm)", "Window Title"="FOFB - Gráfico BPMs Horizontais", "BPM?"=TRUE, "Monitoring Queue Name"="BPM Horizontal Monitoring Data" ("Window Title"), "Selected Readings"=w320, "Variable Names"=w322) -> ()  [unwired: 7 in, 2 out]
                        }
                      }
                    }
                    frame 1 {
                      n159 = case shown="True" w333 {
                        tunnel: w334 -> [_ w343]
                        tunnel: w332 -> [_ _]
                        tunnel: w331 -> [_ w336]
                        frame False {
                        }
                        frame True {
                          w338 = 25
                          n160 = for {
                            N: w338 -> [_]
                            tunnel: w338 -> [w346]
                            tunnel: [w344] -> w337 mode=indexing
                            i -> [w345]
                            n161 = Add(x=w346, y=w345) -> (x+y=w344:i32)
                          }
                          n162 = for {
                            tunnel: w336 -> [w347]
                            tunnel: w337 -> [w349] mode=indexing
                            tunnel: [w348] -> w339 mode=indexing
                            n163 = Index Array(array=w347, index=w349) -> (element=w348:string)
                          }
                          n164 = call-by-ref "Start Asynchronous Call"(reference=w343, "Graph Unit"="Amplitude (mm)", "Window Title"="FOFB - Gráfico BPMs Verticais", "BPM?"=TRUE, "Monitoring Queue Name"="BPM Vertical Monitoring Data" ("Window Title"), "Selected Readings"=w337, "Variable Names"=w339) -> ()  [unwired: 7 in, 2 out]
                        }
                      }
                    }
                  }
                }
              }
            }
            n165 = invoke class="VI" method="FP.Close"(reference=w255) -> ()  [unwired: 2 in, 3 out]
          }
          event "Open Computer Performance": Value Change {
            n166 = event-data() -> ("NewVal"=w352:bool)  [unwired: 1 in, 4 out]
            n167 = case shown="True" w352 {
              frame False {
              }
              frame True {
                n168 = vi-ref "GUI Controller Performace Window.vi"() -> (w359:refnum<vi>)
                n169 = invoke class="VI" method="FP.Open"(reference=w359, "Activate"=TRUE ("Activate?"), "State"=T7."Standard") -> (reference out=w353:refnum<vi>, error out=w358:errorcluster)  [unwired: 2 in, 3 out]
                n170 = call <vilib>:"Clear Errors.vi"("error in (no error)"=w358) -> ("error out"=w355:errorcluster)  [unwired: 6 in]
                n171 = invoke class="VI" method="Run VI"(reference=w353, error in=w355, "Wait until done"=FALSE ("Wait Until Done"), "Auto Dispose Ref"=FALSE ("Auto Dispose Reference")) -> (error out=w354:errorcluster)  [unwired: 1 in, 4 out]
                n172 = call <vilib>:"Clear Errors.vi"("error in (no error)"=w354) -> ()  [unwired: 6 in, 1 out]
              }
            }
          }
        }
        n173 = Unbundle By Name(w109) -> ("Stop VIs Notifier"=w108:refnum<notifier>)
        n174 = flat-sequence {
          tunnel: w112 -> [w118]
          tunnel: w108 -> [w121]
          tunnel: [w120] -> w110
          tunnel: [w118] -> w111
          frame #0 {
            n175 = Wait on Notification(notifier=w121, timeout in ms (-1)=0) -> (notification=w120:bool)  [unwired: 2 in, 3 out]
          }
        }
        n176 = node-c288() -> ()  [unwired: 1 in, 1 out]
      }
      n177 = timed-loop {
        timing: w76 -> [_]
        timing-out: [_] -> w75
        tunnel: w52 -> [w93]
        tunnel: w51 -> [w90]
        shift-right: [w89] -> w19
        shift-left: w12 -> [w88]
        stop <- w92 stop-if-true
        n178 = node-c288() -> ()  [unwired: 1 in, 1 out]
        n179 = Dequeue Element(queue=w93, timeout in ms (-1)=0, error in (no error)=w88) -> (element=w96:bool, timed out?=w95:bool, error out=w91:errorcluster)  [unwired: 1 out]
        n180 = case shown="False" w95 {
          tunnel: w96 -> [w101 _]
          frame False {
            "Connected" <- w101
          }
          frame True {
          }
        }
        n181 = flat-sequence {
          tunnel: [w100] -> w89
          tunnel: w91 -> [w100]
          tunnel: w90 -> [w99]
          tunnel: [w98] -> w92
          frame #0 {
            n182 = Wait on Notification(notifier=w99, timeout in ms (-1)=0) -> (notification=w98:bool)  [unwired: 2 in, 3 out]
          }
        }
        n183 = node-c288() -> ()  [unwired: 1 in, 1 out]
      }
      n184 = call "GUI Monitoring Loop.vi"("error in (no error)"=w12, "Sync Objects"=w10, "FOFB Parameters"=w15) -> ("error out"=w67:errorcluster)  [unwired: 8 in]
      n185 = call "GUI Configuration Loop.vi"("FOFB Controller IP"=w14, "error in (no error)"=w12, "FOFB GUI"=w10, "TCP Listening Timeout"=1000 ("timeout ms (60000)"), "Configuration GUI TCP Port"=u16 3602 ("remote port or service name")) -> ("error out"=w66:errorcluster)  [unwired: 6 in]
      n186 = node-c288(w75) -> ()  [unwired: 1 out]
      n187 = Unbundle By Name(w10) -> ("RMS Monitoring Data Queue"=w56:refnum<queue>, "BPM / PS Monitoring Data Notifiers"=w47:refnum<queue>[], "Performance Monitoring Data Notifier"=w41:refnum<queue>)
      n188 = node-c288(w81) -> ()  [unwired: 1 out]
      n189 = Index Array(array=w47) -> (element #1=w46:refnum<queue>, element #2=w45:refnum<queue>, element #3=w44:refnum<queue>, element #4=w43:refnum<queue>, element #5=w42:refnum<queue>)  [unwired: 5 in]
      n190 = timed-loop "User interface update loop" {
        tunnel: w58 -> [w433]
        shift-right: [w421] -> w68
        shift-left: w12 -> [w432]
        border: w60 -> [_]
        tunnel: w57 -> [w430]
        tunnel: w63 -> [w423]
        tunnel: w62 -> [w422]
        tunnel: w51 -> [w420]
        tunnel: w56 -> [w417]
        timing: w80 -> [_]
        timing-out: [_] -> w79
        tunnel: w50 -> [w412]
        tunnel: w49 -> [w411]
        tunnel: w48 -> [w410]
        tunnel: w46 -> [w403]
        tunnel: w45 -> [w402]
        tunnel: w44 -> [w401]
        tunnel: w43 -> [w400]
        tunnel: w42 -> [w399]
        tunnel: w41 -> [w398]
        tunnel: w33 -> [w389]
        shift-right: [w369] -> w27
        shift-left: _ -> [w376]
        shift-right: [w370] -> _
        shift-left: _ -> [w378]
        tunnel: w25 -> [w375]
        stop <- w364 stop-if-true
        w406 = T22 {"Timestamp"=timestamp(0 s since 1904-01-01), "Sample"=[]} ("Monitoring Sample")
        # "### Operation mode name translation"
        n191 = node-c288() -> ()  [unwired: 1 in, 1 out]
        n192 = feedback #2(u32 0 ("Number of Averages")) -> (w373:u32)
        n193 = Less Or Equal To 0?(x=w373) -> (x <= 0?=w368:bool)
        n194 = case shown="True" w368 {
          tunnel: [w442 w451] -> w379
          tunnel: w378 -> [w442 _]
          tunnel: [w441 w450] -> w377
          tunnel: w376 -> [w441 w449]
          tunnel: w375 -> [_ w444]
          tunnel: w373 -> [w440 _]
          tunnel: [w439 u32 12000 ("Number of Averages")] -> w367
          frame False {
            n195 = Decrement(x=w440) -> (x-1=w439:u32)
          }
          frame True {
            # "###"
            n196 = Get Date/Time In Seconds() -> (seconds since 1Jan1904=w447:timestamp)
            n197 = Format Date/Time String(time format string (%c)="%Y.%m.%d-%Hh%Mm%S%3u.tdms", seconds (now)=w447) -> (date/time string=w445:string)  [unwired: 1 in]
            n198 = Build Path(base path=w444, name or relative path=w445) -> (appended path=w453:path)
            n199 = TDMS Open(7:enum16{"1.0", "2.0"}."1.0" ("file format version (2.0)"), 8:w449, 10:T13."create or replace" ("operation (0:open)"), 11:w453) -> (0:w450:errorcluster, 3:w451:refnum<k34>)  [unwired: 2 in]
          }
        }
        n200 = feedback-in #2(w367) -> ()
        n201 = Dequeue Element(queue=w433, timeout in ms (-1)=-1, error in (no error)=w432) -> (element=w397:T23, error out=w418:errorcluster)  [unwired: 2 out]
        n202 = Unbundle By Name(w397) -> ("BPM Readings"=w387:dbl[], "Diagnostics Data"=w395:T10, "PS Readings"=w408:dbl[], "PS FOFB Setpoints"=w409:dbl[], "Timestamp"=w384:timestamp, "Operation Mode"=w394:T24)
        n203 = Wait on Notification(notifier=w430, timeout in ms (-1)=0) -> (notification=w427:dbl[])  [unwired: 2 in, 3 out]
        n204 = First Call?() -> (First Call?: T/F=w413:bool)
        n205 = call "MultiChannel Moving Average Filter PtByPt.vi"("Initialize"=w413, "Number of Averages"=w423, "X"=w387) -> ("Filtered X"=w388:dbl[])  [unwired: 8 in]
        n206 = Array Size(array=w427) -> (size(s)=w428:i32)
        n207 = case shown="\"FOFB Mode\"" w394 {
          tunnel: [T1."Corr. órbita via OPR1" ("Operation Mode (Controller to GUI)") T1."Corr. órbita via FOFB" ("Operation Mode (Controller to GUI)") T1."Medida de Matriz Resposta" ("Operation Mode (Controller to GUI)")] -> w416
          frame "Manual Mode", Default {
          }
          frame "FOFB Mode" {
          }
          frame "RMM Mode" {
          }
        }
        "Operation Mode (Controller to GUI)" <- w416
        n208 = call "MultiChannel Moving Average Filter PtByPt.vi"("Initialize"=w413, "Number of Averages"=u32 100, "X"=w388) -> ("Filtered X"=→"Current Orbit":dbl[])  [unwired: 8 in]
        n209 = feedback #3() -> (w429:dbl[])
        n210 = case shown="1, Default" w428 {
          tunnel: w427 -> [_ w518]
          tunnel: w429 -> [w517 _]
          tunnel: [w517 w518] -> w396
          frame 0 {
          }
          frame 1, Default {
          }
        }
        "Reference Orbit" <- w396
        n211 = feedback-in #3(w396) -> ()
        n212 = Subtract(x=w396, y=w388) -> (x-y=w390:dbl[])
        n213 = feedback #4() -> (w424:u32)  [unwired: 1 in]
        n214 = Equal?(x=w422, y=w424) -> (x = y?=w426:bool)
        n215 = case shown="True" w426 {
          tunnel: w424 -> [w461 _]
          tunnel: [w460 u32 0] -> w425
          tunnel: w412 -> [_ w482]
          tunnel: w411 -> [_ w478]
          tunnel: w390 -> [_ w473]
          tunnel: w410 -> [_ w472]
          frame False {
            n216 = Increment(x=w461) -> (x+1=w460:u32)
          }
          frame True {
            n217 = Split 1D Array(array=w473, index=w472) -> (first subarray=w469:dbl[], second subarray=w471:dbl[])
            n218 = for {
              tunnel: [w516] -> w474 mode=indexing
              tunnel: w469 -> [w514] mode=indexing
              i -> [w515]
              n219 = Bundle(w515, w514) -> (w516:cluster{i32, dbl})  [unwired: 1 in]
            }
            "Horizontal" <- w474
            n220 = for {
              tunnel: w471 -> [w511] mode=indexing
              tunnel: [w513] -> w475 mode=indexing
              i -> [w512]
              n221 = Bundle(w512, w511) -> (w513:cluster{i32, dbl})  [unwired: 1 in]
            }
            "Vertical" <- w475
            n222 = call-poly <vilib>:"RMS.vi"("X"=w469) -> ("rms value"=→"RMS X":dbl)  [unwired: 1 out]
            n223 = call-poly <vilib>:"RMS.vi"("X"=w471) -> ("rms value"=→"RMS Y":dbl)  [unwired: 1 out]
            n224 = Absolute Value(x=w469) -> (abs(x)=w487:dbl[])
            n225 = Absolute Value(x=w471) -> (abs(x)=w483:dbl[])
            n226 = Array Max & Min(array=w487) -> (max value=w463:dbl, max index (indices)=w486:i32, min index (indices)=w468:i32)  [unwired: 1 out]
            n227 = Array Max & Min(array=w483) -> (max value=w462:dbl, max index (indices)=w466:i32, min index (indices)=w467:i32)  [unwired: 1 out]
            n228 = Index Array(array=w482, index #1=w486, index #2=w468) -> (element #1=→"Max X @":string, element #2=→"Min X @":string)
            n229 = Index Array(array=w469, index #1=w486, index #2=w468) -> (element #1=→"Max. X":dbl, element #2=→"Min X":dbl)
            n230 = Index Array(array=w471, index #1=w466, index #2=w467) -> (element #1=→"Max. Y":dbl, element #2=→"Min Y":dbl)
            n231 = Index Array(array=w478, index #1=w466, index #2=w467) -> (element #1=→"MaxY @":string, element #2=→"Min Y @":string)
            n232 = flat-sequence {
              tunnel: "Auto-Scale" -> [w492]
              tunnel: w463 -> [w491]
              tunnel: w462 -> [w490]
              frame #0 {
                n233 = case shown="True" w492 {
                  tunnel: w491 -> [_ w503]
                  tunnel: w490 -> [_ w495]
                  frame False {
                  }
                  frame True {
                    w497 = 10.0 ("y")
                    w493 = 1.2 ("x")
                    w504 = 10.0 ("y")
                    n234 = Multiply(x=w503, y=w504) -> (x*y=w506:dbl)
                    n235 = Multiply(x=w495, y=w497) -> (x*y=w499:dbl)
                    n236 = Round Toward +Infinity(x=w506) -> (ceil(x): smallest int >= x=w505:dbl)
                    n237 = Round Toward +Infinity(x=w499) -> (ceil(x): smallest int >= x=w498:dbl)
                    n238 = Divide(x=w505, y=w504) -> (x/y=w501:dbl)
                    n239 = Divide(x=w498, y=w497) -> (x/y=w496:dbl)
                    n240 = Multiply(x=w493, y=w501) -> (x*y=w500:dbl)
                    n241 = Multiply(x=w493, y=w496) -> (x*y=w494:dbl)
                    n242 = property on="Max Scale X" class="DigNum (strict)"("Value"=w500) -> ()  [unwired: 2 in, 2 out]
                    n243 = property on="Max Scale Y" class="DigNum (strict)"("Value"=w494) -> ()  [unwired: 2 in, 2 out]
                    n244 = property on="Auto-Scale" class="Bool (strict)"("Value"=FALSE) -> ()  [unwired: 2 in, 2 out]
                  }
                }
              }
              frame #1 {
                n245 = Negate(x="Max Scale X") -> (-x=w510:dbl)
                n246 = Negate(x="Max Scale Y") -> (-x=w508:dbl)
                n247 = property on="Horizontal" class="XYGraph (strict)"("YScale.Maximum"="Max Scale X") -> ()  [unwired: 2 in, 2 out]
                n248 = property on="Horizontal" class="XYGraph (strict)"("YScale.Minimum"=w510) -> ()  [unwired: 2 in, 2 out]
                n249 = property on="Vertical" class="XYGraph (strict)"("YScale.Maximum"="Max Scale Y") -> ()  [unwired: 2 in, 2 out]
                n250 = property on="Vertical" class="XYGraph (strict)"("YScale.Minimum"=w508) -> ()  [unwired: 2 in, 2 out]
              }
            }
          }
        }
        n251 = feedback-in #4(w425) -> ()
        n252 = Seconds To Date/Time(time stamp (now)=w384) -> (date time rec=w386:T25)  [unwired: 1 in]
        n253 = Date/Time To Seconds(1:TRUE ("is UTC (F)"), 2:w386) -> (0:w383:timestamp)
        n254 = To Double Precision Float(number=w383) -> (double precision float=w382:dbl)
        n255 = Build Array (concatenate)(w408, w409) -> (w391:dbl[])
        n256 = Bundle By Name(cluster=w406, "Timestamp"=w384, "Sample"=w390) -> (w393:T22)
        n257 = Lossy Enqueue Element(queue=w417, element=w393) -> ()  [unwired: 1 in, 4 out]
        n258 = Lossy Enqueue Element(queue=w403, element=w393) -> ()  [unwired: 1 in, 4 out]
        n259 = Bundle By Name(cluster=T9 {"Timestamp"=timestamp(0 s since 1904-01-01), "Diagnostics Data"={"Time-Critical Loop Missed Iterations"=0, "Time-Critical Loop Execution Time (usec)"=0, "FA Buffer Usage"=0, "Available Memory (bytes)"=0, "CPU Loads Array"=[]}} ("Diagnostics  Sample"), "Diagnostics Data"=w395, "Timestamp"=w384) -> (w405:T9)
        n260 = Lossy Enqueue Element(queue=w402, element=w393) -> ()  [unwired: 1 in, 4 out]
        n261 = Bundle By Name(cluster=w406, "Sample"=w391, "Timestamp"=w384) -> (w407:T22)
        n262 = Lossy Enqueue Element(queue=w401, element=w407) -> ()  [unwired: 1 in, 4 out]
        n263 = Build Array (concatenate)(w382, w387, w391) -> (w380:dbl[])
        n264 = Lossy Enqueue Element(queue=w400, element=w407) -> ()  [unwired: 1 in, 4 out]
        n265 = Lossy Enqueue Element(queue=w399, element=w407) -> ()  [unwired: 1 in, 4 out]
        n266 = flat-sequence {
          tunnel: [w459] -> w421
          tunnel: w418 -> [w459]
          tunnel: w420 -> [w458]
          tunnel: [w457] -> w364
          frame #0 {
            n267 = Wait on Notification(notifier=w458, timeout in ms (-1)=0) -> (notification=w457:bool)  [unwired: 2 in, 3 out]
          }
        }
        n268 = Lossy Enqueue Element(queue=w398, element=w405) -> ()  [unwired: 1 in, 4 out]
        n269 = TDMS Write(0:w379, 1:enum16{"decimated", "interleaved"}."interleaved" ("data layout (0:decimated)"), 5:"FOFB BPM and PS Monitoring Data" ("group name in (Untitled)"), 7:w389, 9:w380, 11:w377) -> (4:w371:refnum<k34>, 15:w372:errorcluster)  [unwired: 2 out]
        n270 = Less Or Equal To 0?(x=w367) -> (x <= 0?=w366:bool)
        n271 = Compound Arithmetic op=OR(w366, w364) -> (w365:bool)
        n272 = case shown="True" w365 {
          tunnel: w372 -> [w434 w438]
          tunnel: w371 -> [w435 w437]
          tunnel: [w435 _] -> w370
          tunnel: [w434 w436] -> w369
          frame False {
          }
          frame True {
            n273 = TDMS Close(8:w438, 11:w437) -> (0:w436:errorcluster)  [unwired: 1 out]
          }
        }
        n274 = node-c288() -> ()  [unwired: 1 in, 1 out]
      }
      n275 = node-c288(w77) -> ()  [unwired: 1 out]
      n276 = Close Reference(reference=w55) -> (error out=w53:errorcluster)  [unwired: 1 in]
      n277 = node-c288(w79) -> ()  [unwired: 1 out]
      n278 = Merge Errors(w53, w69, w66, w67, w19, w27, w68) -> (w54:errorcluster)
      n279 = call "GUI Close Synchronization Objects.vi"("error in (no error)"=w54, "FOFB GUI"=w10) -> ("error out"=→"error out":errorcluster)  [unwired: 9 in]
    }
    frame True {
    }
  }
